vi "Factorial.vi"(3 "n":i32) -> (1 "n!":dbl format="%.2f")   [LabVIEW 2017, in "NI_Gmath.lvlib"]
doc: "Computes the factorial of <B>n</B>."
uses:
  <vilib>/gmath/NI_Gmath.lvlib
  <resource>/lvanlys.dll
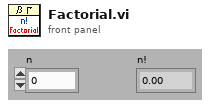
[diagram p1: front panel]
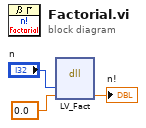
[diagram p0: block diagram]
diagram:
  n1 = dll-call lib="e:/builds/penguin/labview/branches/2017/dev/dist/resource/lvanlys.*" fn="LV_Fact"("n"="n", "n!"=0.0 ("factorial")) -> ("n!"=→"n!":dbl)  [unwired: 5 in, 2 out]
